vi "Connect.vi"(6 "Timeout (ms)":i32=5000, 7 "Cache Symbols?(T)":bool, 8 "error in (no error)":errorcluster, 9 "Port":i32=851, 10 "Net ID":string) -> (0 "error out":errorcluster, 3 "TwinCAT ADS out":refnum<class "TwinCAT ADS.lvclass">)   [LabVIEW 2018, in "TwinCAT ADS.lvclass"]
uses:
  TwinCAT ADS.lvclass
  TwinCAT ADS.lvclass/TwinCAT ADS.ctl
  TwinCAT.Ads
panel:
  in  "TwinCAT ADS in":refnum<class "TwinCAT ADS.lvclass">
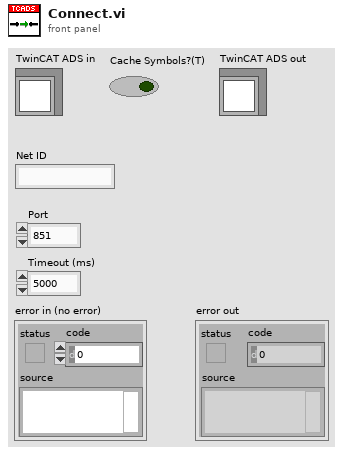
[diagram p1: front panel]
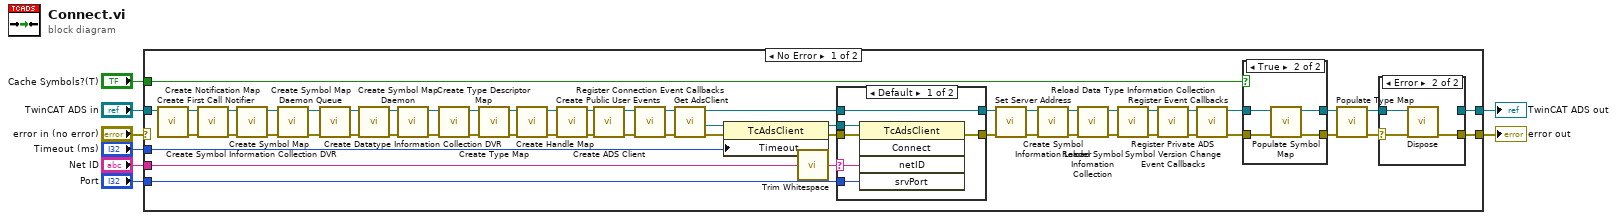
[diagram p0: block diagram]
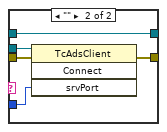
[diagram p4: hidden frame]
diagram:
  n1 = case shown="No Error" "error in (no error)" {
    selector: "error in (no error)" -> [_ w88]
    tunnel: [w31 w88] -> w7
    tunnel: [w32 w87] -> w5
    tunnel: "TwinCAT ADS in" -> [w22 w87]
    tunnel: "Net ID" -> [w64 _]
    tunnel: "Port" -> [w65 _]
    tunnel: "Timeout (ms)" -> [w54 _]
    tunnel: "Cache Symbols?(T)" -> [w13 _]
    frame No Error {
      n2 = call "Create First Call Notifier.vi"("TwinCAT ADS in"=w22) -> ("error out"=w20:errorcluster, "TwinCAT ADS out"=w21:refnum<class "TwinCAT ADS.lvclass">)  [unwired: 9 in]
      n3 = call "Create Notification Map.vi"("error in (no error)"=w20, "TwinCAT ADS in"=w21) -> ("error out"=w29:errorcluster, "TwinCAT ADS out"=w30:refnum<class "TwinCAT ADS.lvclass">)  [unwired: 8 in]
      n4 = call "Create Symbol Information Collection DVR.vi"("error in (no error)"=w29, "TwinCAT ADS in"=w30) -> ("error out"=w33:errorcluster, "TwinCAT ADS out"=w34:refnum<class "TwinCAT ADS.lvclass">)  [unwired: 8 in]
      n5 = call "Create Symbol Map.vi"("error in (no error)"=w33, "TwinCAT ADS in"=w34) -> ("error out"=w18:errorcluster, "TwinCAT ADS out"=w19:refnum<class "TwinCAT ADS.lvclass">)  [unwired: 8 in]
      n6 = call "Create Symbol Map Daemon Queue.vi"("error in (no error)"=w18, "TwinCAT ADS in"=w19) -> ("error out"=w14:errorcluster, "TwinCAT ADS out"=w17:refnum<class "TwinCAT ADS.lvclass">)  [unwired: 8 in]
      n7 = call "Create Symbol Map Daemon.vi"("error in (no error)"=w14, "TwinCAT ADS in"=w17) -> ("error out"=w15:errorcluster, "TwinCAT ADS out"=w16:refnum<class "TwinCAT ADS.lvclass">)  [unwired: 8 in]
      n8 = call "Create Datatype Information Collection DVR.vi"("error in (no error)"=w15, "TwinCAT ADS in"=w16) -> ("error out"=w11:errorcluster, "TwinCAT ADS out"=w12:refnum<class "TwinCAT ADS.lvclass">)  [unwired: 8 in]
      n9 = call "Create Type Descriptor Map.vi"("error in (no error)"=w11, "TwinCAT ADS in"=w12) -> ("error out"=w9:errorcluster, "TwinCAT ADS out"=w10:refnum<class "TwinCAT ADS.lvclass">)  [unwired: 8 in]
      n10 = call "Create Type Map.vi"("error in (no error)"=w9, "TwinCAT ADS in"=w10) -> ("error out"=w43:errorcluster, "TwinCAT ADS out"=w46:refnum<class "TwinCAT ADS.lvclass">)  [unwired: 8 in]
      n11 = call "Create Handle Map.vi"("error in (no error)"=w43, "TwinCAT ADS in"=w46) -> ("error out"=w44:errorcluster, "TwinCAT ADS out"=w45:refnum<class "TwinCAT ADS.lvclass">)  [unwired: 8 in]
      n12 = call "Create Public User Events.vi"("error in (no error)"=w44, "TwinCAT ADS in"=w45) -> ("error out"=w48:errorcluster, "TwinCAT ADS out"=w49:refnum<class "TwinCAT ADS.lvclass">)  [unwired: 8 in]
      n13 = call "Create ADS Client.vi"("error in (no error)"=w48, "TwinCAT ADS in"=w49) -> ("error out"=w52:errorcluster, "TwinCAT ADS out"=w53:refnum<class "TwinCAT ADS.lvclass">)  [unwired: 8 in]
      n14 = call "Register Connection Event Callbacks.vi"("error in (no error)"=w52, "TwinCAT ADS in"=w53) -> ("error out"=w51:errorcluster, "TwinCAT ADS out"=w50:refnum<class "TwinCAT ADS.lvclass">)  [unwired: 8 in]
      n15 = call "Get AdsClient.vi"("error in (no error)"=w51, "TwinCAT ADS in"=w50) -> ("error out"=w57:errorcluster, ".NET TcAdsClient"=w56:refnum<k24>, "TwinCAT ADS out"=w55:refnum<class "TwinCAT ADS.lvclass">)  [unwired: 7 in]
      n16 = property class="TcAdsClient"(reference=w56, error in=w57, "Timeout"=w54) -> (reference out=w62:refnum<k24>, error out=w63:errorcluster)
      n17 = call <vilib>:"Trim Whitespace.vi"("string"=w64) -> ("trimmed string"=w59:string)  [unwired: 1 in]
      n18 = case shown="Default" w59 {
        selector: w59 -> [w77 _]
        tunnel: w63 -> [w81 w86]
        tunnel: w65 -> [w80 w83]
        tunnel: w62 -> [w79 w85]
        tunnel: [w78 w84] -> w58
        tunnel: w55 -> [w76 w82]
        tunnel: [w76 w82] -> w47
        frame Default {
          n19 = invoke class="TcAdsClient" method="Connect"(reference=w79, error in=w81, "netID"=w77, "srvPort"=w80) -> (error out=w78:errorcluster)  [unwired: 1 in, 4 out]
        }
        frame "" {
          n20 = invoke class="TcAdsClient" method="Connect"(reference=w85, error in=w86, "srvPort"=w83) -> (error out=w84:errorcluster)  [unwired: 1 in, 3 out]
        }
      }
      n21 = call "Set Server Address.vi"("error in (no error)"=w58, "TwinCAT ADS in"=w47) -> ("error out"=w37:errorcluster, "TwinCAT ADS out"=w38:refnum<class "TwinCAT ADS.lvclass">)  [unwired: 8 in]
      n22 = call "Create Symbol Information Loader.vi"("error in (no error)"=w37, "TwinCAT ADS in"=w38) -> ("error out"=w36:errorcluster, "TwinCAT ADS out"=w35:refnum<class "TwinCAT ADS.lvclass">)  [unwired: 8 in]
      n23 = call "Reload Symbol Infomation Collection.vi"("error in (no error)"=w36, "TwinCAT ADS in"=w35) -> ("error out"=w60:errorcluster, "TwinCAT ADS out"=w61:refnum<class "TwinCAT ADS.lvclass">)  [unwired: 8 in]
      n24 = call "Reload Data Type Information Collection.vi"("error in (no error)"=w60, "TwinCAT ADS in"=w61) -> ("error out"=w42:errorcluster, "TwinCAT ADS out"=w41:refnum<class "TwinCAT ADS.lvclass">)  [unwired: 8 in]
      n25 = call "Register Private ADS Symbol Version Change Event Callbacks.vi"("error in (no error)"=w42, "TwinCAT ADS in"=w41) -> ("error out"=w39:errorcluster, "TwinCAT ADS out"=w40:refnum<class "TwinCAT ADS.lvclass">)  [unwired: 8 in]
      n26 = call "Register Event Callbacks.vi"("error in (no error)"=w39, "TwinCAT ADS in"=w40) -> ("error out"=w26:errorcluster, "TwinCAT ADS out"=w28:refnum<class "TwinCAT ADS.lvclass">)  [unwired: 8 in]
      n27 = case shown="True" w13 {
        tunnel: w28 -> [w66 w71]
        tunnel: [w66 w70] -> w27
        tunnel: w26 -> [w67 w69]
        tunnel: [w67 w68] -> w25
        frame False {
        }
        frame True {
          n28 = call "Populate Symbol Map.vi"("error in (no error)"=w69, "TwinCAT ADS in"=w71) -> ("error out"=w68:errorcluster, "TwinCAT ADS out"=w70:refnum<class "TwinCAT ADS.lvclass">)  [unwired: 8 in]
        }
      }
      n29 = call "Populate Type Map.vi"("error in (no error)"=w25, "TwinCAT ADS in"=w27) -> ("error out"=w23:errorcluster, "TwinCAT ADS out"=w24:refnum<class "TwinCAT ADS.lvclass">)  [unwired: 8 in]
      n30 = case shown="Error" w23 {
        selector: w23 -> [_ w75]
        tunnel: w24 -> [w72 w74]
        tunnel: [w72 _] -> w32
        tunnel: [_ w73] -> w31
        frame No Error {
        }
        frame Error {
          n31 = call "Dispose.vi"("error in (no error)"=w75, "TwinCAT ADS in"=w74) -> ("error out"=w73:errorcluster)  [unwired: 9 in]
        }
      }
    }
    frame Error {
    }
  }
  "error out" <- w7
  "TwinCAT ADS out" <- w5
